vi "hamilton_controller.vi"(6 "VISA resource name in":refnum<visa-resource-name>, 8 "error in":errorcluster, 9 "Open?":bool, 10 "valve":enum16{"A", "B", "ALL"}(ring), 11 "action":T1(ring)) -> (0 "error out":errorcluster, 2 "VISA resource name out":refnum<visa-resource-name>)   [LabVIEW 2014]
uses:
  <vilib>/Instr/_visa.llb/VISA Configure Serial Port (Instr).vi
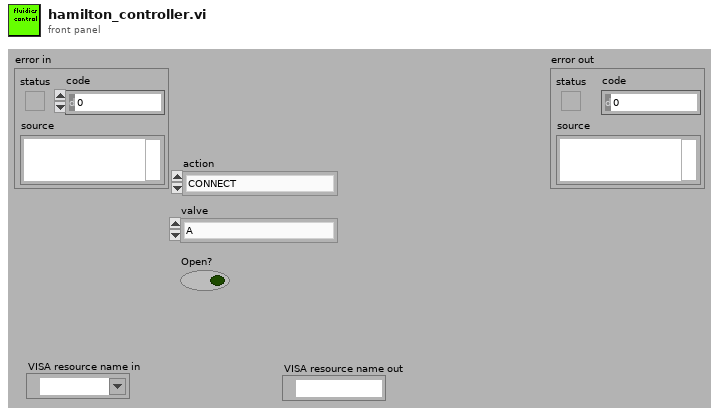
[diagram p1: front panel]
types:
  T1 = enum16{"CONNECT", "INITIALIZE VALVES", "DISCONNECT", "MOVE VALVE"}
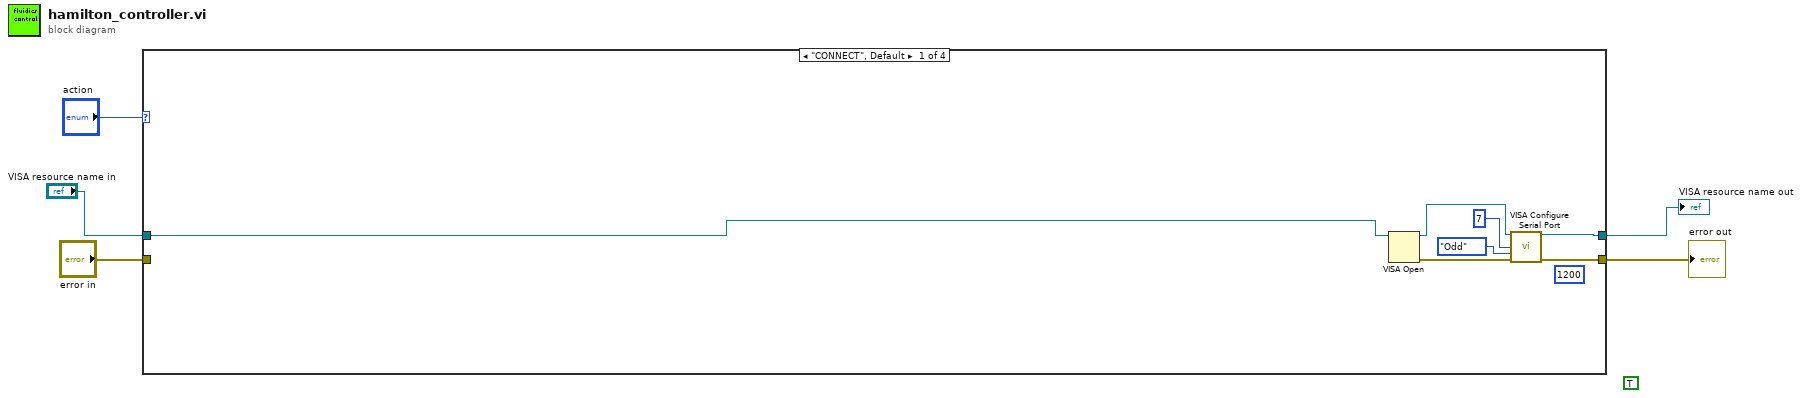
[diagram p0: block diagram]
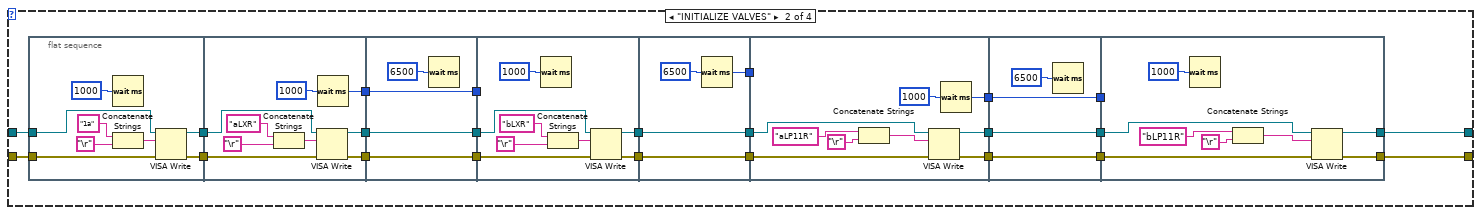
[diagram p2: hidden frame]
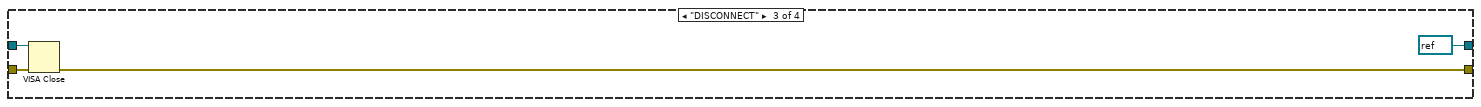
[diagram p3: hidden frame]
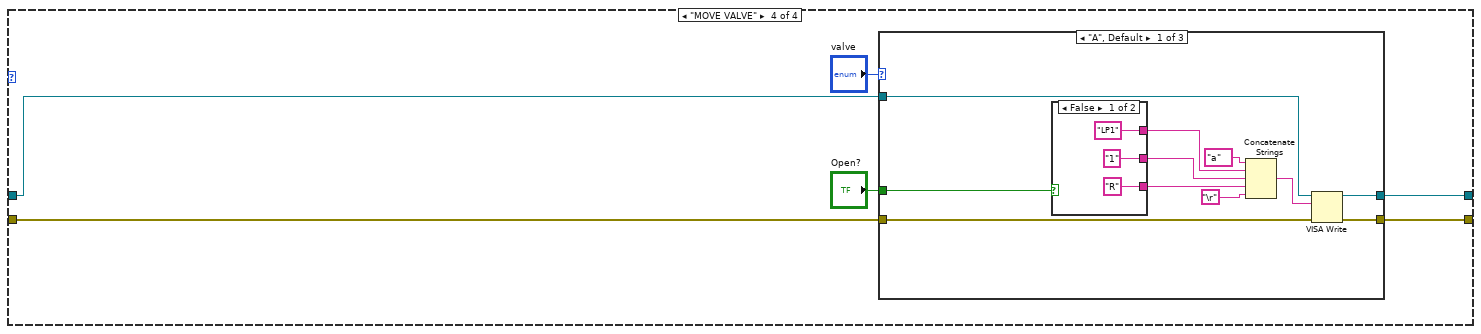
[diagram p4: hidden frame]
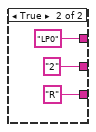
[diagram p5: hidden frame]
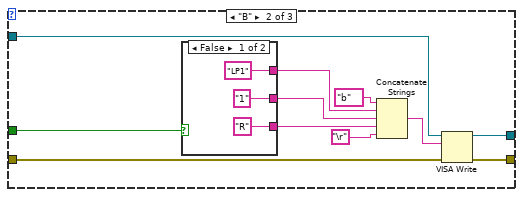
[diagram p6: hidden frame]
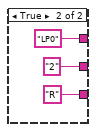
[diagram p7: hidden frame]
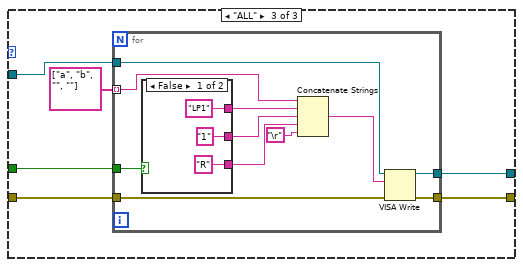
[diagram p8: hidden frame]
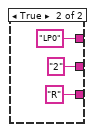
[diagram p9: hidden frame]
diagram:
  (unwired) TRUE
  n1 = case shown="\"CONNECT\", Default" "action" {
    tunnel: [w8 w14 refnum<visa-resource-name> refnum ("VISA resource name out") w96] -> w1
    tunnel: [w7 w13 w91 w95] -> w3
    tunnel: "VISA resource name in" -> [w6 w30 w93 w98]
    tunnel: "error in" -> [_ w29 w92 w97]
    frame "CONNECT", Default {
      (unwired) u32 1200 ("baud rate (9600)")
      n2 = VISA Open(VISA resource name=w6) -> (VISA resource name=w12:refnum<visa-resource-name>, error out=w9:errorcluster)  [unwired: 4 in]
      n3 = call-poly "VISA Configure Serial Port"("VISA resource name"=w12, "data bits (8)"=u16 7, "parity (0:none)"=enum16{"None", "Odd", "Even", "Mark", "Space"}."Odd", "error in (no error)"=w9) -> ("VISA resource name out"=w8:refnum<visa-resource-name>, "error out"=w7:errorcluster)  [unwired: 10 in]
    }
    frame "INITIALIZE VALVES" {
      n4 = flat-sequence {
        tunnel: w30 -> [w43]
        tunnel: w29 -> [w42]
        tunnel: [w41] -> w35
        tunnel: [w37] -> w34
        tunnel: w35 -> [w51]
        tunnel: w34 -> [w52]
        tunnel: [w50] -> w28
        tunnel: [w45] -> w26
        tunnel: [w44] -> w24
        tunnel: w28 -> [w56]
        tunnel: [w56] -> w27
        tunnel: w26 -> [w55]
        tunnel: [w55] -> w25
        tunnel: w24 -> [w54]
        tunnel: [w54] -> w23
        tunnel: w27 -> [_]
        tunnel: w25 -> [w64]
        tunnel: w23 -> [w63]
        tunnel: [w58] -> w16
        tunnel: [w57] -> w15
        tunnel: [w66] -> w33
        tunnel: [w67] -> w32
        tunnel: [w65] -> w31
        tunnel: w16 -> [w66]
        tunnel: w15 -> [w65]
        tunnel: w33 -> [w71]
        tunnel: w32 -> [_]
        tunnel: w31 -> [w69]
        tunnel: [w74] -> w22
        tunnel: [w72] -> w20
        tunnel: [w70] -> w18
        tunnel: w22 -> [w81]
        tunnel: [w81] -> w21
        tunnel: w20 -> [w80]
        tunnel: [w80] -> w19
        tunnel: w18 -> [w79]
        tunnel: [w79] -> w17
        tunnel: w21 -> [w85]
        tunnel: w19 -> [_]
        tunnel: w17 -> [w84]
        tunnel: [w83] -> w14
        tunnel: [w82] -> w13
        frame #0 {
          n5 = Wait (ms)(milliseconds to wait=u32 1000) -> ()  [unwired: 1 out]
          n6 = Concatenate Strings("1a" ("string"), "\r") -> (w38:string)
          n7 = VISA Write(VISA resource name=w43, write buffer=w38, error in (no error)=w42) -> (VISA resource name out=w37:refnum<visa-resource-name>, error out=w41:errorcluster)  [unwired: 1 out]
        }
        frame #1 {
          n8 = Concatenate Strings("aLXR", "\r") -> (w46:string)
          n9 = VISA Write(VISA resource name=w52, write buffer=w46, error in (no error)=w51) -> (VISA resource name out=w45:refnum<visa-resource-name>, error out=w44:errorcluster)  [unwired: 1 out]
          n10 = Wait (ms)(milliseconds to wait=u32 1000) -> (millisecond timer value=w50:u32)
        }
        frame #2 {
          n11 = Wait (ms)(milliseconds to wait=u32 6500) -> ()  [unwired: 1 out]
        }
        frame #3 {
          n12 = Wait (ms)(milliseconds to wait=u32 1000) -> ()  [unwired: 1 out]
          n13 = Concatenate Strings("bLXR", "\r") -> (w59:string)
          n14 = VISA Write(VISA resource name=w64, write buffer=w59, error in (no error)=w63) -> (VISA resource name out=w58:refnum<visa-resource-name>, error out=w57:errorcluster)  [unwired: 1 out]
        }
        frame #4 {
          n15 = Wait (ms)(milliseconds to wait=u32 6500) -> (millisecond timer value=w67:u32)
        }
        frame #5 {
          n16 = Concatenate Strings("aLP11R" ("string"), "\r") -> (w77:string)
          n17 = VISA Write(VISA resource name=w71, write buffer=w77, error in (no error)=w69) -> (VISA resource name out=w70:refnum<visa-resource-name>, error out=w74:errorcluster)  [unwired: 1 out]
          n18 = Wait (ms)(milliseconds to wait=u32 1000) -> (millisecond timer value=w72:u32)
        }
        frame #6 {
          n19 = Wait (ms)(milliseconds to wait=u32 6500) -> ()  [unwired: 1 out]
        }
        frame #7 {
          n20 = Wait (ms)(milliseconds to wait=u32 1000) -> ()  [unwired: 1 out]
          n21 = Concatenate Strings("bLP11R" ("string"), "\r") -> (w89:string)
          n22 = VISA Write(VISA resource name=w84, write buffer=w89, error in (no error)=w85) -> (VISA resource name out=w83:refnum<visa-resource-name>, error out=w82:errorcluster)  [unwired: 1 out]
        }
      }
    }
    frame "DISCONNECT" {
      n23 = VISA Close(VISA resource name=w93, error in (no error)=w92) -> (error out=w91:errorcluster)
    }
    frame "MOVE VALVE" {
      n24 = case shown="\"A\", Default" "valve" {
        tunnel: w98 -> [w104 w121 w139]
        tunnel: w97 -> [w103 w120 w136]
        tunnel: [w102 w119 w134] -> w96
        tunnel: [w101 w118 w135] -> w95
        tunnel: "Open?" -> [w100 w117 w138]
        frame "A", Default {
          n25 = case shown="False" w100 {
            tunnel: ["R" "R"] -> w108
            tunnel: ["1" "2"] -> w109
            tunnel: ["LP1" ("string") "LP0" ("string")] -> w106
            frame False {
            }
            frame True {
            }
          }
          n26 = Concatenate Strings("a" ("MVP ID"), w106, w109, w108, "\r") -> (w105:string)
          n27 = VISA Write(VISA resource name=w104, write buffer=w105, error in (no error)=w103) -> (VISA resource name out=w102:refnum<visa-resource-name>, error out=w101:errorcluster)  [unwired: 1 out]
        }
        frame "B" {
          n28 = case shown="False" w117 {
            tunnel: ["R" "R"] -> w125
            tunnel: ["1" "2"] -> w126
            tunnel: ["LP1" ("string") "LP0" ("string")] -> w123
            frame False {
            }
            frame True {
            }
          }
          n29 = Concatenate Strings("b" ("MVP ID"), w123, w126, w125, "\r") -> (w122:string)
          n30 = VISA Write(VISA resource name=w121, write buffer=w122, error in (no error)=w120) -> (VISA resource name out=w119:refnum<visa-resource-name>, error out=w118:errorcluster)  [unwired: 1 out]
        }
        frame "ALL" {
          n31 = for {
            tunnel: w139 -> [w146]
            tunnel: w138 -> [w145]
            tunnel: string[] ["a", "b", "", ""] -> [w144] mode=indexing
            tunnel: w136 -> [w142]
            tunnel: [w141] -> w135
            tunnel: [w140] -> w134
            n32 = case shown="False" w145 {
              tunnel: ["R" "R"] -> w149
              tunnel: ["1" "2"] -> w150
              tunnel: ["LP1" ("string") "LP0" ("string")] -> w147
              frame False {
              }
              frame True {
              }
            }
            n33 = Concatenate Strings(w144, w147, w150, w149, "\r") -> (w143:string)
            n34 = VISA Write(VISA resource name=w146, write buffer=w143, error in (no error)=w142) -> (VISA resource name out=w140:refnum<visa-resource-name>, error out=w141:errorcluster)  [unwired: 1 out]
          }
        }
      }
    }
  }
  "error out" <- w3
  "VISA resource name out" <- w1
